vi "Master Setup Read Write References.vi"(0 "Master Exited (in)":refnum<vi>, 1 "Read (F)/ Write (T)":bool, 5 "Master Open (in)":refnum<vi>, 7 "Master Save (in)":refnum<vi>, 9 "Update Channels (in)":refnum<vi>, 11 "Update Channel Rings (in)":refnum<vi>) -> (4 "Master Exited (out)":refnum<vi>, 6 "Master Open (out)":refnum<vi>, 8 "Master Save (out)":refnum<vi>, 10 "Update Channels (out)":refnum<vi>, 14 "Valid References":bool, 15 "Update Channel Rings (out)":refnum<vi>)   [LabVIEW 2017]
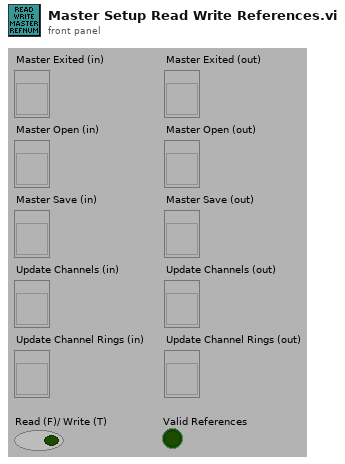
[diagram p1: front panel]
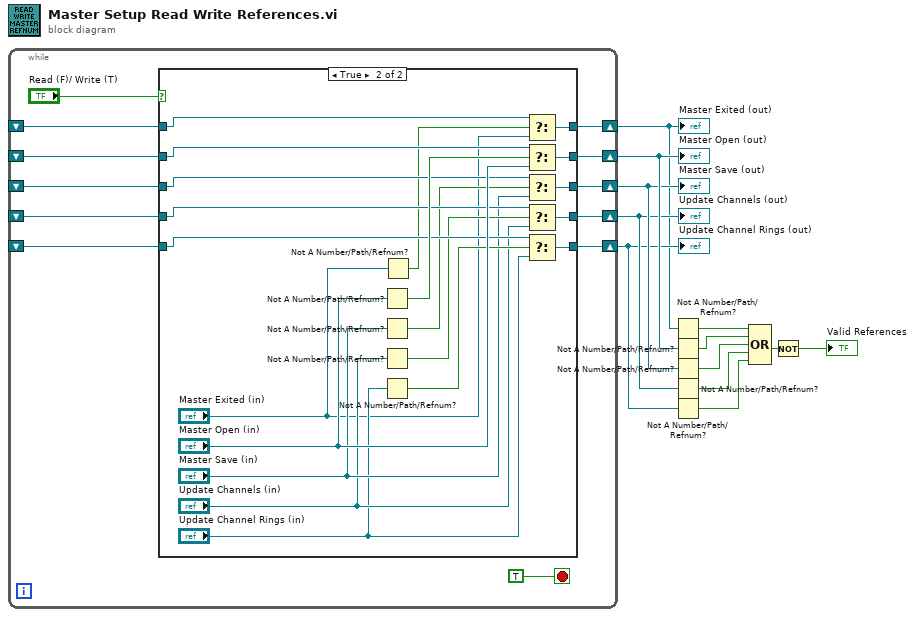
[diagram p0: block diagram]
diagram:
  n1 = while {
    shift-right: [w24] -> w12
    shift-left: _ -> [w19]
    shift-right: [w23] -> w11
    shift-left: _ -> [w18]
    shift-right: [w22] -> w10
    shift-left: _ -> [w17]
    shift-right: [w21] -> w9
    shift-left: _ -> [w16]
    shift-right: [w14] -> w1
    shift-left: _ -> [w13]
    stop <- TRUE stop-if-true
    n2 = case shown="True" "Read (F)/ Write (T)" {
      tunnel: [w29 w46] -> w24
      tunnel: [w28 w45] -> w23
      tunnel: [w27 w44] -> w22
      tunnel: [w26 w43] -> w21
      tunnel: w19 -> [w29 w47]
      tunnel: w18 -> [w28 w42]
      tunnel: w17 -> [w27 w41]
      tunnel: w16 -> [w26 w40]
      tunnel: [w25 w33] -> w14
      tunnel: w13 -> [w25 w30]
      frame False {
      }
      frame True {
        n3 = Not A Number/Path/Refnum?(number/path/refnum="Master Open (in)") -> (NaN/Path/Refnum?=w49:bool)
        n4 = Not A Number/Path/Refnum?(number/path/refnum="Master Save (in)") -> (NaN/Path/Refnum?=w39:bool)
        n5 = Not A Number/Path/Refnum?(number/path/refnum="Update Channels (in)") -> (NaN/Path/Refnum?=w37:bool)
        n6 = Not A Number/Path/Refnum?(number/path/refnum="Update Channel Rings (in)") -> (NaN/Path/Refnum?=w38:bool)
        n7 = Not A Number/Path/Refnum?(number/path/refnum="Master Exited (in)") -> (NaN/Path/Refnum?=w31:bool)
        n8 = Select(t=w30, s=w31, f="Master Exited (in)") -> (s? t:f=w33:refnum<vi>)
        n9 = Select(t=w47, s=w49, f="Master Open (in)") -> (s? t:f=w46:refnum<vi>)
        n10 = Select(t=w42, s=w39, f="Master Save (in)") -> (s? t:f=w45:refnum<vi>)
        n11 = Select(t=w41, s=w37, f="Update Channels (in)") -> (s? t:f=w44:refnum<vi>)
        n12 = Select(t=w40, s=w38, f="Update Channel Rings (in)") -> (s? t:f=w43:refnum<vi>)
      }
    }
  }
  "Master Open (out)" <- w12
  "Master Save (out)" <- w11
  "Update Channel Rings (out)" <- w9
  "Update Channels (out)" <- w10
  "Master Exited (out)" <- w1
  n13 = Not A Number/Path/Refnum?(number/path/refnum=w1) -> (NaN/Path/Refnum?=w2:bool)
  n14 = Not A Number/Path/Refnum?(number/path/refnum=w12) -> (NaN/Path/Refnum?=w8:bool)
  n15 = Not A Number/Path/Refnum?(number/path/refnum=w11) -> (NaN/Path/Refnum?=w7:bool)
  n16 = Not A Number/Path/Refnum?(number/path/refnum=w10) -> (NaN/Path/Refnum?=w6:bool)
  n17 = Not A Number/Path/Refnum?(number/path/refnum=w9) -> (NaN/Path/Refnum?=w5:bool)
  n18 = Compound Arithmetic op=OR(w2, w8, w7, w6, w5) -> (w4:bool)
  n19 = Not(x=w4) -> (.not. x?=→"Valid References":bool)
